vi "Gen position coords array.vi"(8 "Error in":errorcluster, 10 "Number of rows to generate":i32=6, 11 "Experiment Parameters":T1={"Total Number of Miniscans"=1012, "Number of Trials"=20, "Number of cycles in a trial"=344, "Number of miniscans in a frame (Y)"=44, "Number of Pixels in Miniscan (X)"=85, "Number of Frames in Each Trial"=7912, "Number of Frames in a Cycle"=23, "DwellTime (us)"=0.05, "Acquisition length (sec)"=10.0, "Variable Length"=FALSE, "Pixels in miniscan (X)"=[], "Number of lines in frame (Y)"=[]}) -> (0 "error out":errorcluster, 3 "Coordinates of montage positions":cluster{"X\n\nY":i32[]}[](array[cluster]))   [LabVIEW 2020]
uses:
  Typedefs/Experiment Parameters.ctl
panel:
  out "Number of columns to generate":i32
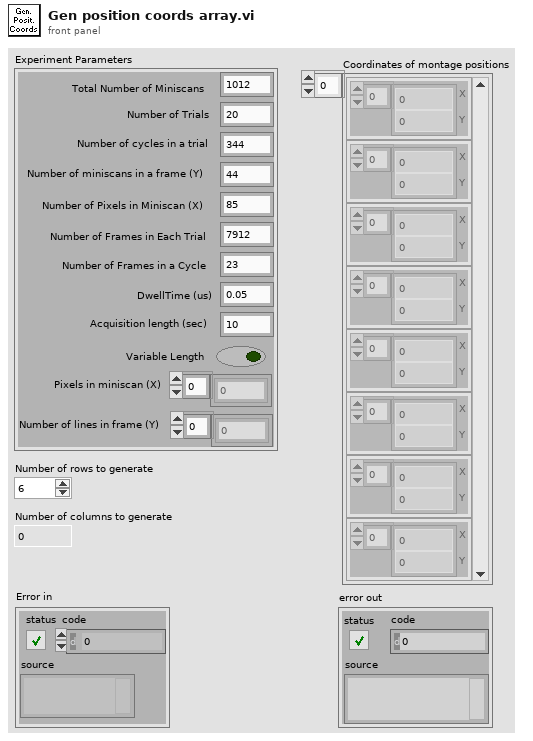
[diagram p1: front panel]
types:
  T1 = typedef "Experiment Parameters.ctl" = cluster{"Total Number of Miniscans":i32, "Number of Trials":i32, "Number of cycles in a trial":i32, "Number of miniscans in a frame (Y)":i32, "Number of Pixels in Miniscan (X)":i32, "Number of Frames in Each Trial":i32, "Number of Frames in a Cycle":i32, "DwellTime (us)":dbl, "Acquisition length (sec)":dbl, "Variable Length":bool, "Pixels in miniscan (X)":dbl[], "Number of lines in frame (Y)":dbl[]}
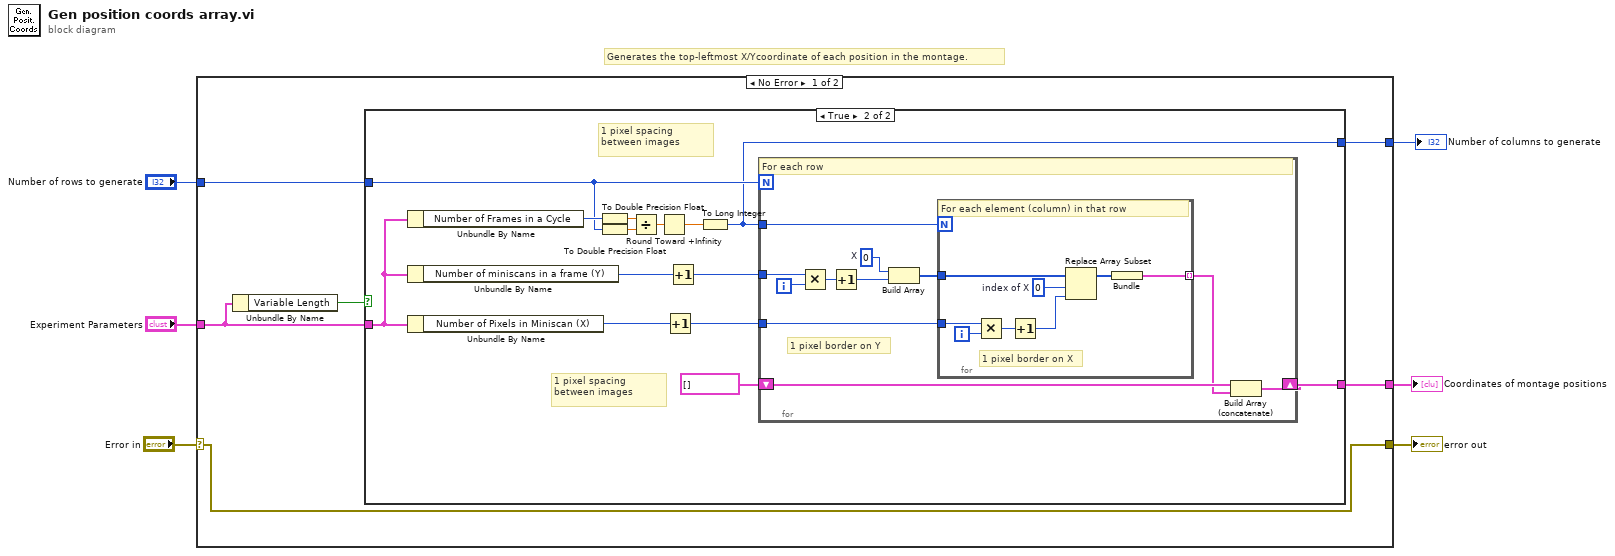
[diagram p0: block diagram]
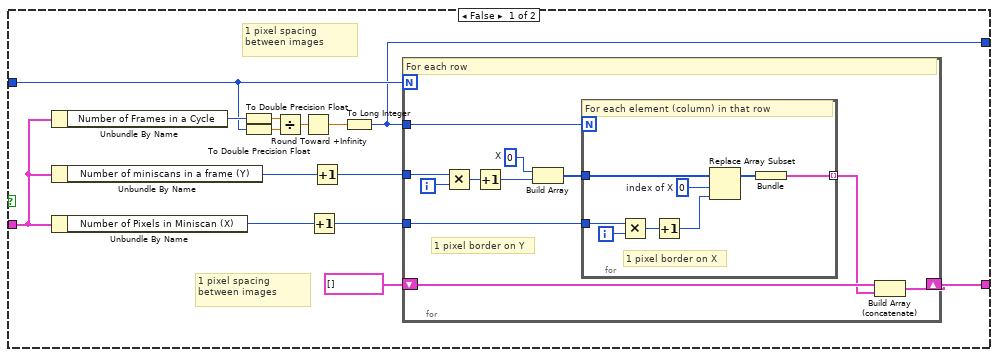
[diagram p2: hidden frame]
diagram:
  # "Generates the top-leftmost X/Ycoordinate of each position in the montage."
  n1 = case shown="No Error" "Error in" {
    selector: "Error in" -> [w10 w79]
    tunnel: "Experiment Parameters" -> [w8 _]
    tunnel: "Number of rows to generate" -> [w12 _]
    tunnel: [w11 _] -> w4
    tunnel: [w10 w79] -> w2
    tunnel: [w9 _] -> w1
    frame No Error {
      n2 = Unbundle By Name(w8) -> ("Variable Length"=w7:bool)
      n3 = case shown="True" w7 {
        tunnel: w8 -> [w21 w54]
        tunnel: w12 -> [w20 w53]
        tunnel: [w16 w49] -> w11
        tunnel: [w15 w48] -> w9
        frame False {
          # "1 pixel spacing between images"
          # "1 pixel spacing between images"
          n4 = Unbundle By Name(w21) -> ("Number of Frames in a Cycle"=w25:i32)
          n5 = Unbundle By Name(w21) -> ("Number of miniscans in a frame (Y)"=w19:i32)
          n6 = Unbundle By Name(w21) -> ("Number of Pixels in Miniscan (X)"=w18:i32)
          n7 = To Double Precision Float(number=w25) -> (double precision float=w23:dbl)
          n8 = To Double Precision Float(number=w20) -> (double precision float=w22:dbl)
          n9 = Divide(x=w23, y=w22) -> (x/y=w24:dbl)
          n10 = Round Toward +Infinity(x=w24) -> (ceil(x): smallest int >= x=w26:dbl)
          n11 = Increment(x=w18) -> (x+1=w13:i32)
          n12 = Increment(x=w19) -> (x+1=w14:i32)
          n13 = To Long Integer(number=w26) -> (32bit integer=w15:i32)
          n14 = for {
            N: w20 -> [_]
            tunnel: w15 -> [w37]
            tunnel: w14 -> [w34]
            tunnel: w13 -> [w31]
            shift-right: [w29] -> w16
            shift-left: cluster{"Offset Left/Top":i32[]}[] [] ("Coordinates of montage positions") -> [w30]
            i -> [w36]
            w32 = 0  # X
            # "1 pixel border on Y"
            # "For each row"
            n15 = Multiply(x=w34, y=w36) -> (x*y=w33:i32)
            n16 = Increment(x=w33) -> (x+1=w27:i32)
            n17 = Build Array(w32, w27) -> (w35:i32[])
            n18 = for {
              N: w37 -> [_]
              tunnel: w35 -> [w45]
              tunnel: w31 -> [w42]
              tunnel: [w39] -> w28 mode=indexing
              i -> [w43]
              w44 = 0  # index of X
              # "1 pixel border on X"
              # "For each element (column) in that row"
              n19 = Multiply(x=w42, y=w43) -> (x*y=w41:i32)
              n20 = Increment(x=w41) -> (x+1=w38:i32)
              n21 = Replace Array Subset "Replace Array Subset"(array=w45, new element=w38, index=w44) -> (w40:i32[])
              n22 = Bundle(w40) -> (w39:cluster{i32[]})  [unwired: 1 in]
            }
            n23 = Build Array (concatenate)(w30, w28) -> (w29:cluster{"Offset Left/Top":i32[]}[])
          }
        }
        frame True {
          # "1 pixel spacing between images"
          # "1 pixel spacing between images"
          n24 = Unbundle By Name(w54) -> ("Number of Frames in a Cycle"=w58:i32)
          n25 = Unbundle By Name(w54) -> ("Number of miniscans in a frame (Y)"=w52:i32)
          n26 = Unbundle By Name(w54) -> ("Number of Pixels in Miniscan (X)"=w51:i32)
          n27 = To Double Precision Float(number=w58) -> (double precision float=w56:dbl)
          n28 = To Double Precision Float(number=w53) -> (double precision float=w55:dbl)
          n29 = Divide(x=w56, y=w55) -> (x/y=w57:dbl)
          n30 = Round Toward +Infinity(x=w57) -> (ceil(x): smallest int >= x=w59:dbl)
          n31 = Increment(x=w51) -> (x+1=w46:i32)
          n32 = Increment(x=w52) -> (x+1=w47:i32)
          n33 = To Long Integer(number=w59) -> (32bit integer=w48:i32)
          n34 = for {
            N: w53 -> [_]
            tunnel: w48 -> [w70]
            tunnel: w47 -> [w67]
            tunnel: w46 -> [w64]
            shift-right: [w62] -> w49
            shift-left: cluster{"Offset Left/Top":i32[]}[] [] ("Coordinates of montage positions") -> [w63]
            i -> [w69]
            w65 = 0  # X
            # "1 pixel border on Y"
            # "For each row"
            n35 = Multiply(x=w67, y=w69) -> (x*y=w66:i32)
            n36 = Increment(x=w66) -> (x+1=w60:i32)
            n37 = Build Array(w65, w60) -> (w68:i32[])
            n38 = for {
              N: w70 -> [_]
              tunnel: w68 -> [w78]
              tunnel: w64 -> [w75]
              tunnel: [w72] -> w61 mode=indexing
              i -> [w76]
              w77 = 0  # index of X
              # "1 pixel border on X"
              # "For each element (column) in that row"
              n39 = Multiply(x=w75, y=w76) -> (x*y=w74:i32)
              n40 = Increment(x=w74) -> (x+1=w71:i32)
              n41 = Replace Array Subset "Replace Array Subset"(array=w78, new element=w71, index=w77) -> (w73:i32[])
              n42 = Bundle(w73) -> (w72:cluster{i32[]})  [unwired: 1 in]
            }
            n43 = Build Array (concatenate)(w63, w61) -> (w62:cluster{"Offset Left/Top":i32[]}[])
          }
        }
      }
    }
    frame Error {
    }
  }
  "Coordinates of montage positions" <- w4
  "error out" <- w2
  "Number of columns to generate" <- w1
